vi "ACK.vi"(8 "error in (no error)":errorcluster, 11 "Instrument in":refnum<class "Instrument.lvclass">) -> (0 "error out":errorcluster, 2 "ACK":string, 3 "Instrument out":refnum<class "Instrument.lvclass">)   [LabVIEW 2019, in "Instrument.lvclass"]
uses:
  Instrument.lvclass
  Typedefs/Instrument.Commands--Enum.ctl
  Instrument.lvclass/Instrument.ctl
  bb8a232c-f628-49fe-96b6-aa36c3f8e839.vi
  bb8a232c-f628-49fe-96b6-aa36c3f8e839.vi/94f5274a-48e1-4e7f-8fad-049fa16a6f23.vi
  Send and Receive.vi
  bb8a232c-f628-49fe-96b6-aa36c3f8e839.vi/94f5274a-48e1-4e7f-8fad-049fa16a6f23.vi/3e6e9521-1bbc-451a-8e8f-81f5580bcc3f.vi
  bb8a232c-f628-49fe-96b6-aa36c3f8e839.vi/94f5274a-48e1-4e7f-8fad-049fa16a6f23.vi/6e128892-7ae8-4983-a850-5ea02fdbae49.vi
  Enum to String.vi
  RemoteControl/API/Send and Receive.vi
  <vilib>/Utility/Data Type/Get Type Information.vi
  <vilib>/JDP Science/JSONtext/JSON text to Variant.vi
  <vilib>/JDP Science/JSONtext/LVClass Serializer/JSONtext LVClass Serializer.lvclass
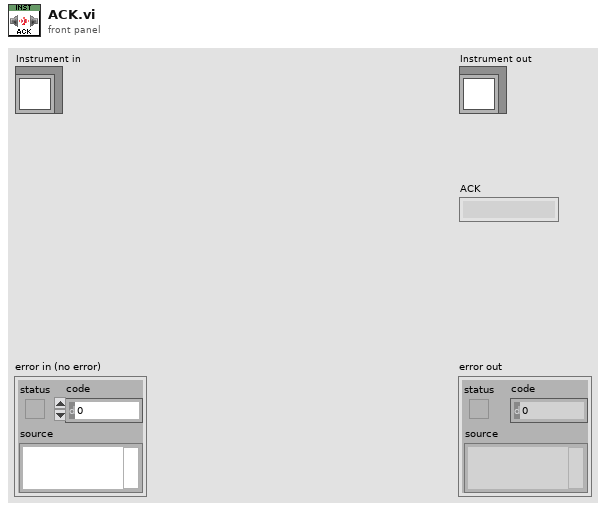
[diagram p1: front panel]
types:
  T1 = typedef "Instrument.lvclass/Instrument.Commands--Enum.ctl" = enum16{"HELP", "ACK", "setConfiguration", "getAll", "getAllData"}
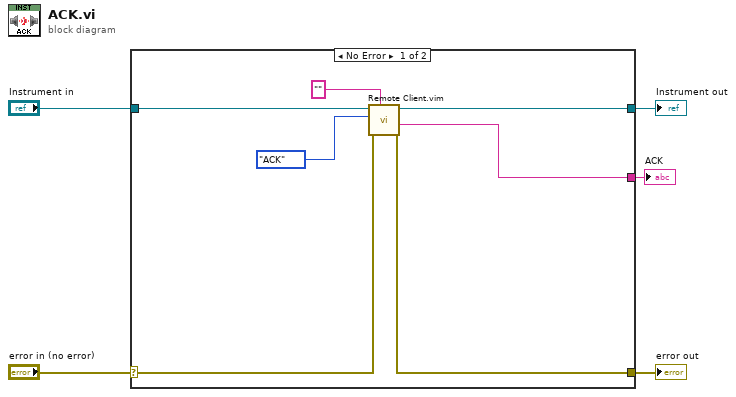
[diagram p0: block diagram]
diagram:
  n1 = case shown="No Error" "error in (no error)" {
    selector: "error in (no error)" -> [w10 w14]
    tunnel: [w7 w14] -> w4
    tunnel: [w12 w13] -> w2
    tunnel: "Instrument in" -> [w11 w13]
    tunnel: [w6 _] -> w1
    frame No Error {
      n2 = call "Remote Client.vim"("Data Out type"="" ("Commands"), "error in (no error)"=w10, "method"=Instrument.Commands--Enum."ACK" ("Commands"), "Instrument in"=w11) -> ("error out"=w7:errorcluster, "Data out"=w6:string, "Instrument out"=w12:refnum<class "Instrument.lvclass">)  [unwired: 4 in, 1 out]
    }
    frame Error {
    }
  }
  "error out" <- w4
  "Instrument out" <- w2
  "ACK" <- w1
